vi "Get Cache.vi"(11 "ConfigManager.Cache in":refnum<class "ConfigManager.Cache.lvclass">) -> (1 "found?":bool, 2 "Cache":refnum<class "ConfigManager.Cache.lvclass">, 3 "ConfigManager.Cache out":refnum<class "ConfigManager.Cache.lvclass">)   [LabVIEW 2013, in "CfgManager.lvlib" / "ConfigManager.Cache.lvclass"]
uses:
  ConfigManager.Cache.lvclass
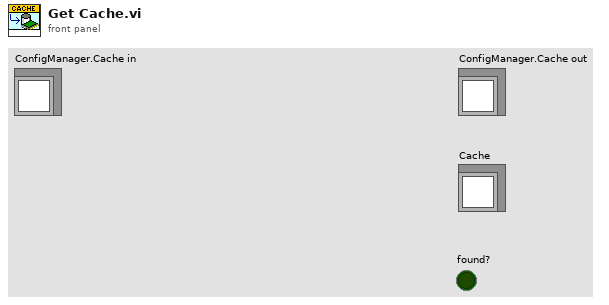
[diagram p1: front panel]
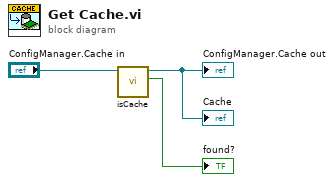
[diagram p0: block diagram]
diagram:
  n1 = call "isCache.vi"("ConfigManager.Cache in"="ConfigManager.Cache in") -> ("isCache?"=→"found?":bool, "ConfigManager.Cache out"=→"ConfigManager.Cache out" →"Cache":refnum<class "ConfigManager.Cache.lvclass">)  [unwired: 9 in]
